vi "Day 9-1.vi"() -> ()   [LabVIEW 2019, in "Day 9.lvlib"]
uses:
  Day 9.lvlib
panel:
  out "numeric array":i32[](array[numeric])
  out "Result":i32
  out "Array":i32[][](array[numeric])
  in  "String":string
  # "477"
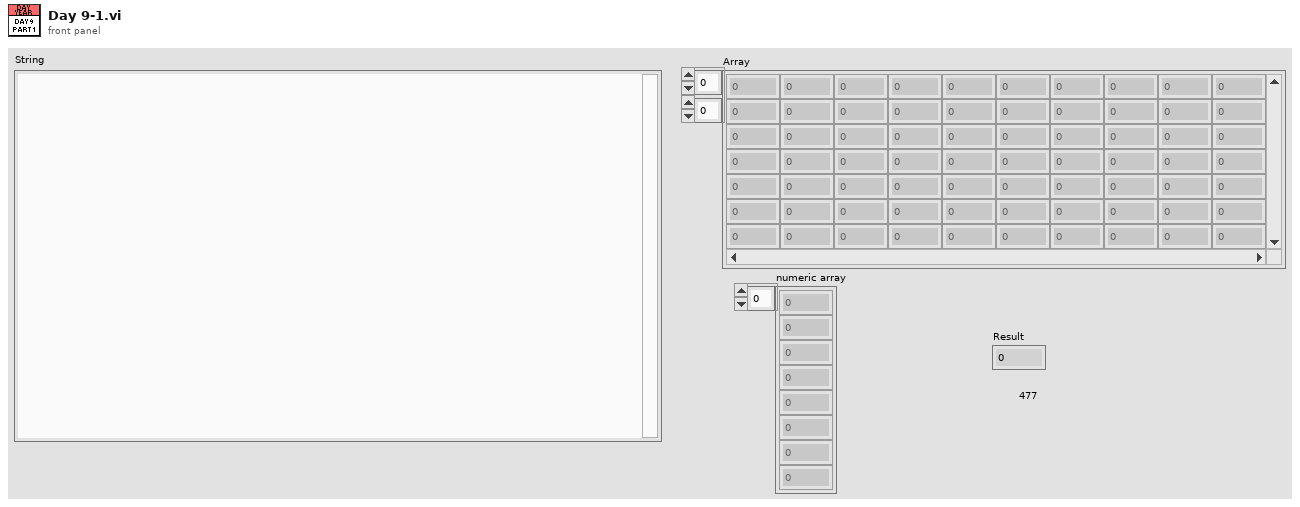
[diagram p1: front panel]
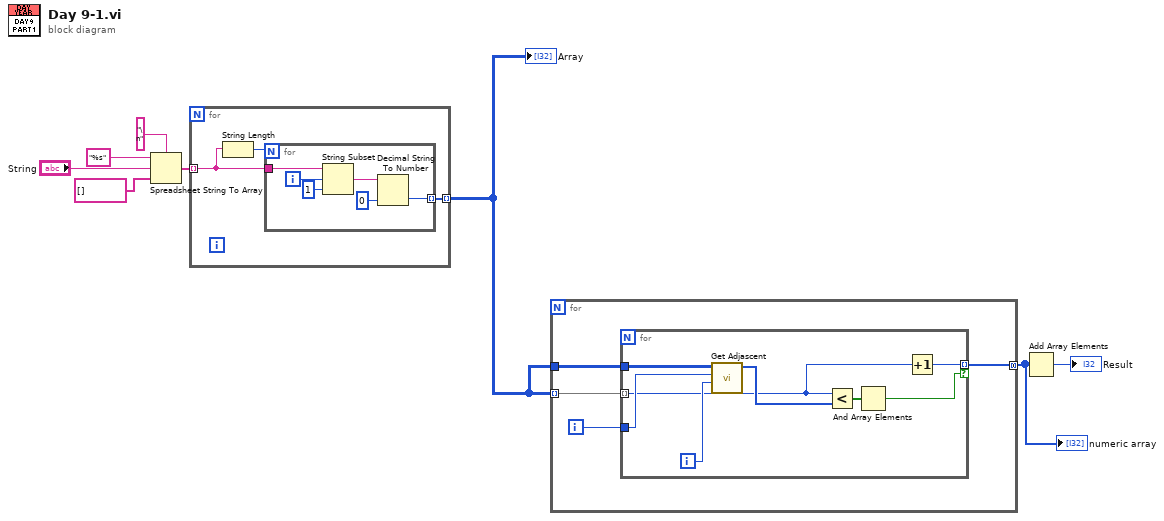
[diagram p0: block diagram]
diagram:
  n1 = Spreadsheet String To Array(delimiter (Tab)="\n", format string="%s", spreadsheet string="String", array type (2D Dbl)=string[] []) -> (array=w4:string[])
  n2 = for {
    tunnel: w4 -> [w11] mode=indexing
    tunnel: [w9] -> w3 mode=indexing
    n3 = String Length(string=w11) -> (length=w10:i32)
    n4 = for {
      N: w10 -> [_]
      tunnel: w11 -> [w17]
      tunnel: [w13] -> w9 mode=indexing
      i -> [w16]
      n5 = String Subset(string=w17, offset (0)=w16, length (rest)=1 ("length (rest)")) -> (substring=w14:string)
      n6 = Decimal String To Number(string=w14, default (0L)=0 ("default (0 I32)")) -> (number=w13:i32)  [unwired: 1 in, 1 out]
    }
  }
  "Array" <- w3
  n7 = for {
    tunnel: w3 -> [w21] mode=indexing
    tunnel: w3 -> [w20]
    tunnel: [w18] -> w1 mode=concatenating
    i -> [w19]
    n8 = for {
      tunnel: w21 -> [w24] mode=indexing
      tunnel: w20 -> [w29]
      tunnel: w19 -> [w27]
      tunnel: [w23] -> w18 mode=indexing if=w22
      i -> [w28]
      n9 = call "Get Adjascent.vi"("column"=w28, "row"=w27, "Array in"=w29) -> ("Array out"=w26:i32[])  [unwired: 8 in]
      n10 = Less?(x=w24, y=w26) -> (x < y?=w25:bool[])
      n11 = And Array Elements(Boolean array=w25) -> (logical AND=w22:bool)
      n12 = Increment(x=w24) -> (x+1=w23:i32)
    }
  }
  "numeric array" <- w1
  n13 = Add Array Elements(numeric array=w1) -> (sum=→"Result":i32)
